vi "Push Buffer to Sink.vi"(8 "error in (no error)":errorcluster, 10 "Log Events":T1[](array[typedef]), 11 "Buffered Log Sink in":refnum<class "Buffered Log Sink.lvclass">) -> (0 "error out":errorcluster, 3 "Buffered Log Sink out":refnum<class "Buffered Log Sink.lvclass">)   [LabVIEW 2019, in "Buffered Log Sink.lvclass"]
uses:
  <vilib>/gpm_packages/@cs/event-logger/Source/Buffered Log Sink/Buffered Log Sink.lvclass
  <vilib>/gpm_packages/@cs/event-logger/Source/Composed Log/Types/Log Packet.ctl
  <vilib>/gpm_packages/@cs/event-logger/Source/Composed Log/Types/Log Level.ctl
  <vilib>/gpm_packages/@cs/event-logger/Source/Buffered Log Sink/Buffered Log Sink.lvclass/Buffered Log Sink.ctl
  <vilib>/gpm_packages/@cs/event-logger/Source/Composed Log/Log Sink/Log Sink.lvclass
  <vilib>/gpm_packages/@cs/event-logger/Source/Composed Log/Composed Log.lvlib
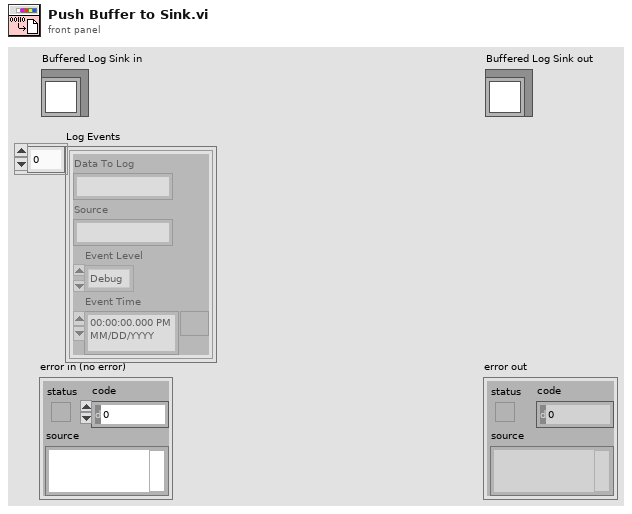
[diagram p1: front panel]
types:
  T1 = typedef "Composed Log.lvlib/Log Packet.ctl" = cluster{"Data To Log":string, "Source":string, "Event Level":T2, "Event Time":timestamp}
  T2 = typedef "Composed Log.lvlib/Log Level.ctl" = enum16{"Debug", "Info", "Warning", "Error", "Critical"}
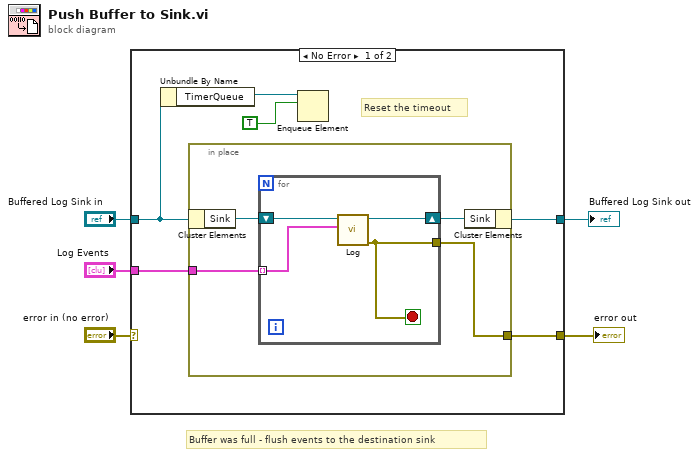
[diagram p0: block diagram]
diagram:
  # "Buffer was full - flush events to the destination sink"
  n1 = case shown="No Error" "error in (no error)" {
    selector: "error in (no error)" -> [_ w20]
    tunnel: "Buffered Log Sink in" -> [w8 w21]
    tunnel: "Log Events" -> [w11 _]
    tunnel: [w10 w21] -> w3
    tunnel: [w9 w20] -> w1
    frame No Error {
      # "Reset the timeout"
      n2 = Unbundle By Name(w8) -> ("TimerQueue"=w7:refnum<queue>)
      n3 = in-place {
        in-place-border: w11 -> [w14]
        in-place-border: [w12] -> w9
        n4 = in-place-cluster #1(w8) -> ("Sink"=w15:refnum<class "Log Sink.lvclass">)
        n5 = for {
          tunnel: w14 -> [w18] mode=indexing
          shift-right: [w17] -> w13
          shift-left: w15 -> [w19]
          tunnel: [w16] -> w12
          stop <- w16 stop-if-true
          n6 = call-dynamic "Log.vi"("Log Packet"=w18, "Log Sink in"=w19) -> ("error out"=w16:errorcluster, "Log Sink out"=w17:refnum<class "Log Sink.lvclass">)  [unwired: 8 in]
        }
        n7 = in-place-cluster #1("Sink"=w13) -> (w10:refnum<class "Buffered Log Sink.lvclass">)
      }
      n8 = Enqueue Element(queue=w7, element=TRUE) -> ()  [unwired: 2 in, 3 out]
    }
    frame Error {
    }
  }
  "error out" <- w1
  "Buffered Log Sink out" <- w3
